vi "Format I2C Data for Display.vi"(0 "user timestamps":T2[](array[typedef]), 5 "timestamp filter":T1[](array[typedef])=[enum."User24", enum."User25", enum."User26", enum."User27", enum."User28", enum."User29", enum."User30", enum."User31"]) -> (4 "display data":string[][](array[string]))   [LabVIEW 2023, in "GettingStarted_Common_148X_Host.lvlib"]
uses:
  GettingStarted_Common_148X_Host.lvlib
  <instrlib>/FlexRIO/CSI-2/v2/FPGA/Types/User Timestamp.ctl
  <instrlib>/FlexRIO/CSI-2/v2/FPGA/Types/Timestamp ID.ctl
  <instrlib>/FlexRIO/CSI-2/v2/FPGA/NI CSI-2 API FPGA v2.lvlib
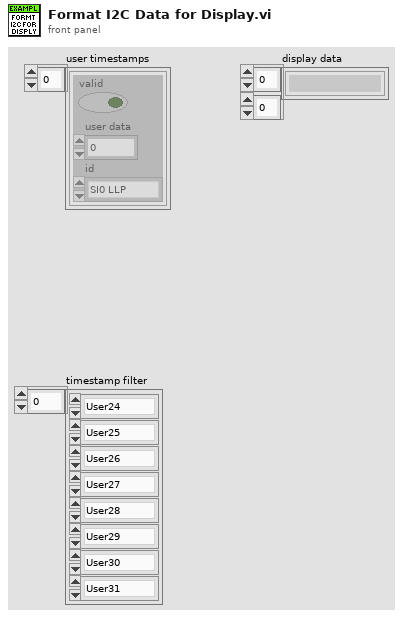
[diagram p1: front panel]
types:
  T1 = typedef "NI CSI-2 API FPGA v2.lvlib/Timestamp ID.ctl" = enum8{"SI0 LLP", "SI1 LLP", "SI2 LLP", "SI3 LLP", "SI4 LLP", "SI5 LLP", "SI6 LLP", "SI7 LLP", "SO0 LLP", "SO1 LLP", "SO2 LLP", "SO3 LLP", "SO4 LLP", "SO5 LLP", "SO6 LLP", "SO7 LLP", "Ser0 GPIO Bank", "Ser1 GPIO Bank", "Ser2 GPIO Bank", "Ser3 GPIO Bank", "Ser4 GPIO Bank", "Ser5 GPIO Bank", "Ser6 GPIO Bank", "Ser7 GPIO Bank", "Des0 GPIO Bank", "Des1 GPIO Bank", "Des2 GPIO Bank", "Des3 GPIO Bank", "Des4 GPIO Bank", "Des5 GPIO Bank", "Des6 GPIO Bank", "Des7 GPIO Bank", "User0", "User1", "User2", "User3", "User4", "User5", "User6", "User7", "User8", "User9", "User10", "User11", "User12", "User13", "User14", "User15", "User16", "User17", "User18", "User19", "User20", "User21", "User22", "User23", "User24", "User25", "User26", "User27", "User28", "User29", "User30", "User31"}
  T2 = typedef "NI CSI-2 API FPGA v2.lvlib/User Timestamp.ctl" = cluster{"valid":bool, "user data":fxp<+,58,58>, "id":T1}
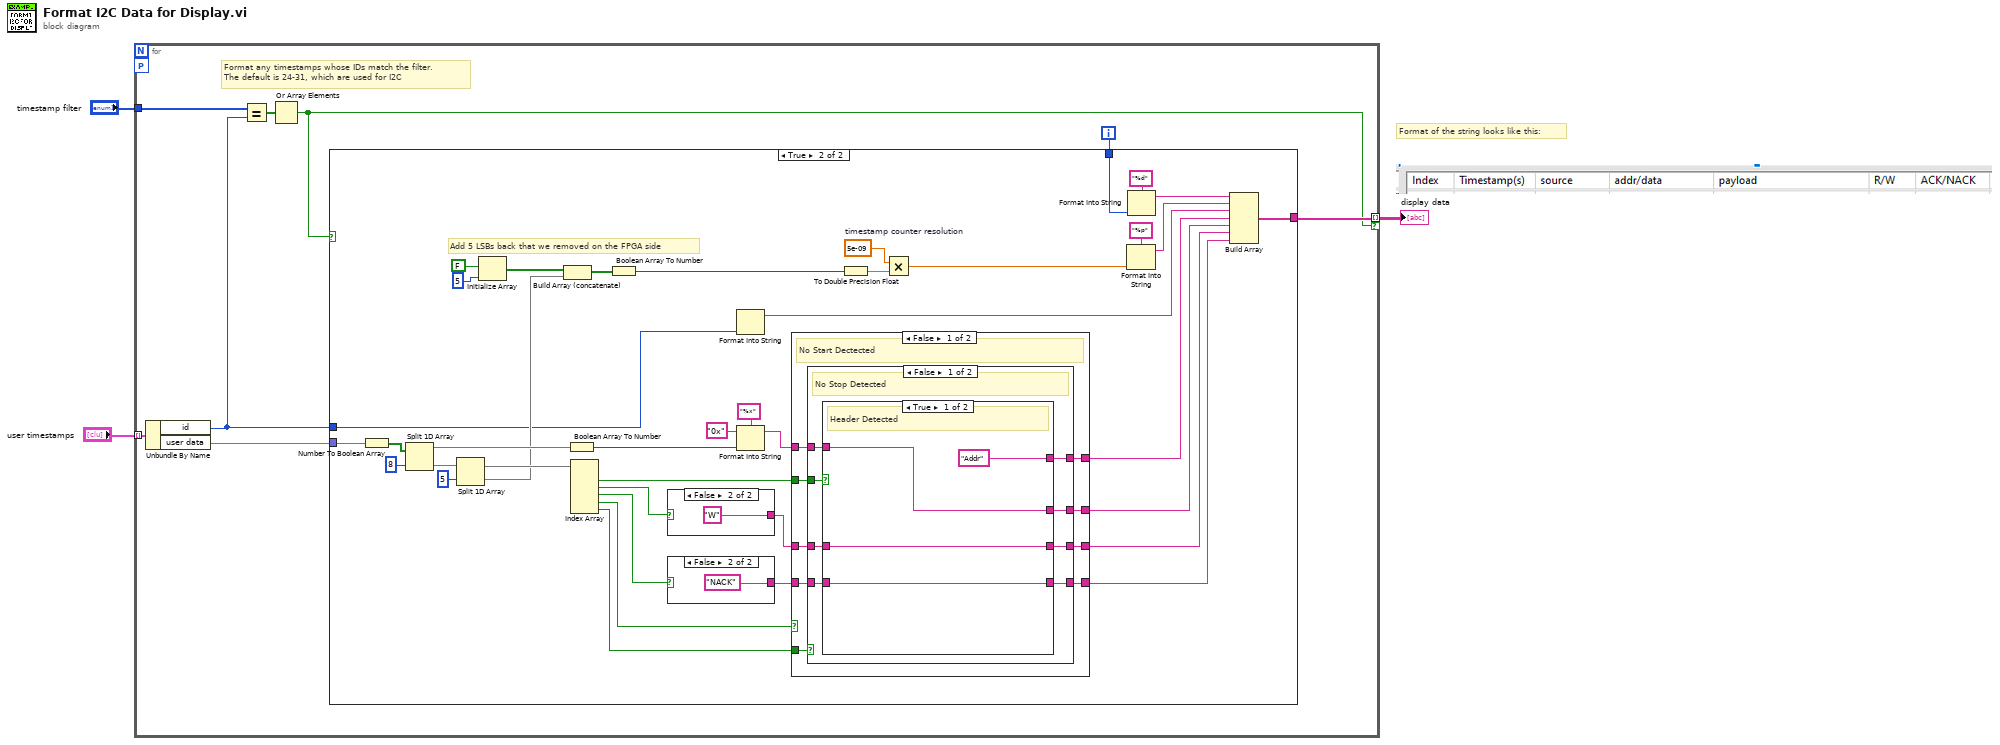
[diagram p0: block diagram]
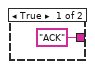
[diagram p3: hidden frame]
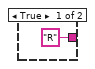
[diagram p4: hidden frame]
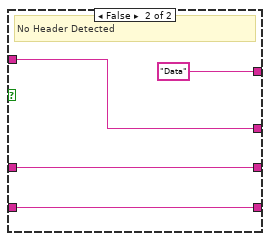
[diagram p5: hidden frame]
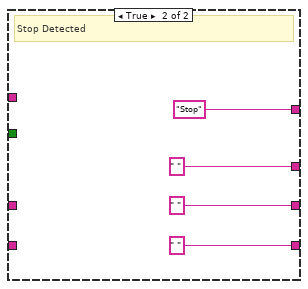
[diagram p6: hidden frame]
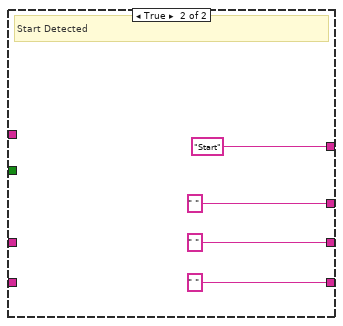
[diagram p7: hidden frame]
diagram:
  # "Format of the string looks like this:"
  n1 = for {
    tunnel: "user timestamps" -> [w11] mode=indexing
    tunnel: [w10] -> w3 mode=indexing if=w4
    workers-P: _ -> [_]
    tunnel: "timestamp filter" -> [w7]
    i -> [w9]
    # "Format any timestamps whose IDs match the filter.\nThe default is 24-31, which are used for I2C"
    n2 = Unbundle By Name(w11) -> ("id"=w5:T1, "user data"=w8:fxp<+,58,58>)
    n3 = Equal?(x=w7, y=w5) -> (x = y?=w6:bool[])
    n4 = Or Array Elements(Boolean array=w6) -> (logical OR=w4:bool)
    n5 = case shown="True" w4 {
      tunnel: [_ w49] -> w10
      tunnel: w9 -> [_ w42]
      tunnel: w8 -> [_ w41]
      tunnel: w5 -> [_ w13]
      frame False {
        # "Do not parse and format timestamps that are not in the timestamp filter"
      }
      frame True {
        w47 = 5e-09  # timestamp counter resolution
        # "Add 5 LSBs back that we removed on the FPGA side"
        n6 = Number To Boolean Array(number=w41) -> (Boolean array=w40:bool[])
        n7 = Split 1D Array(array=w40, index=8) -> (first subarray=w35:bool[], second subarray=w38:bool[])
        n8 = Split 1D Array(array=w38, index=5) -> (first subarray=w36:bool[], second subarray=w31:bool[])
        n9 = Initialize Array(FALSE, 5 ("dimension size")) -> (w32:bool[])
        n10 = Build Array (concatenate)(w32, w31) -> (w30:bool[])
        n11 = Boolean Array To Number(Boolean array=w35) -> (number=w16:u32)
        n12 = Index Array(array=w36) -> (element #1=w26:bool, element #2=w25:bool, element #3=w22:bool, element #4=w28:bool, element #5=w27:bool)  [unwired: 5 in]
        n13 = Boolean Array To Number(Boolean array=w30) -> (number=w29:u64)
        n14 = case shown="False" w25 {
          tunnel: ["R" "W"] -> w24
          frame True {
          }
          frame False {
          }
        }
        n15 = case shown="False" w22 {
          tunnel: ["ACK" "NACK"] -> w23
          frame True {
          }
          frame False {
          }
        }
        n16 = Format Into String(w13) -> (resulting string=w12:string)  [unwired: 3 in, 1 out]
        n17 = Format Into String(format string="%x", initial string="0x", w16) -> (resulting string=w15:string)  [unwired: 1 in, 1 out]
        n18 = case shown="False" w28 {
          tunnel: w27 -> [w63 _]
          tunnel: w26 -> [w62 _]
          tunnel: w24 -> [w61 _]
          tunnel: w23 -> [w60 _]
          tunnel: w15 -> [w59 _]
          tunnel: [w58 "Start"] -> w21
          tunnel: [w57 " "] -> w14
          tunnel: [w56 " "] -> w20
          tunnel: [w55 " "] -> w19
          frame False {
            # "No Start Dectected"
            n19 = case shown="False" w63 {
              tunnel: w62 -> [w71 _]
              tunnel: w61 -> [w70 _]
              tunnel: w60 -> [w69 _]
              tunnel: w59 -> [w68 _]
              tunnel: [w67 "Stop"] -> w58
              tunnel: [w66 " "] -> w57
              tunnel: [w65 " "] -> w56
              tunnel: [w64 " "] -> w55
              frame False {
                # "No Stop Detected"
                n20 = case shown="True" w71 {
                  tunnel: w70 -> [w73 w77]
                  tunnel: w69 -> [w72 w76]
                  tunnel: w68 -> [w74 w78]
                  tunnel: ["Addr" "Data"] -> w67
                  tunnel: [w74 w78] -> w66
                  tunnel: [w73 w77] -> w65
                  tunnel: [w72 w76] -> w64
                  frame True {
                    # "Header Detected"
                  }
                  frame False {
                    # "No Header Detected"
                  }
                }
              }
              frame True {
                # "Stop Detected"
              }
            }
          }
          frame True {
            # "Start Detected"
          }
        }
        n21 = To Double Precision Float(number=w29) -> (double precision float=w46:dbl)
        n22 = Multiply(x=w47, y=w46) -> (x*y=w48:dbl)
        n23 = Format Into String(format string="%p", w48) -> (resulting string=w50:string)  [unwired: 2 in, 1 out]
        n24 = Format Into String(format string="%d", w42) -> (resulting string=w43:string)  [unwired: 2 in, 1 out]
        n25 = Build Array(w43, w50, w12, w21, w14, w20, w19) -> (w49:string[])
      }
    }
  }
  "display data" <- w3
